vi "start_scanning.vi"(8 "error in (no error)":errorcluster, 11 "ScanModeDL090923Scaffold in":refnum<class "ImagingModeDL090923Scaffold.lvclass">) -> (0 "error out":errorcluster, 3 "ScanModeDL090923Scaffold out":refnum<class "ImagingModeDL090923Scaffold.lvclass">)   [LabVIEW 2010, in "ImagingModeDL090923Scaffold.lvclass"]
uses:
  ImagingModeDL090923Scaffold.lvclass
  ImagingModeDL090923Scaffold.lvclass/ImagingModeDL090923Scaffold.ctl
  common/classes/ErrorController/ErrorController/class_data.vi
  ScanHead/GenericScanHead/GenericScanHead/GenericScanHead.lvclass
  DAQ/GenericDAQ/GenericDAQ/GenericDAQ.lvclass
  common/classes/ErrorController/ErrorController/ErrorController.lvclass
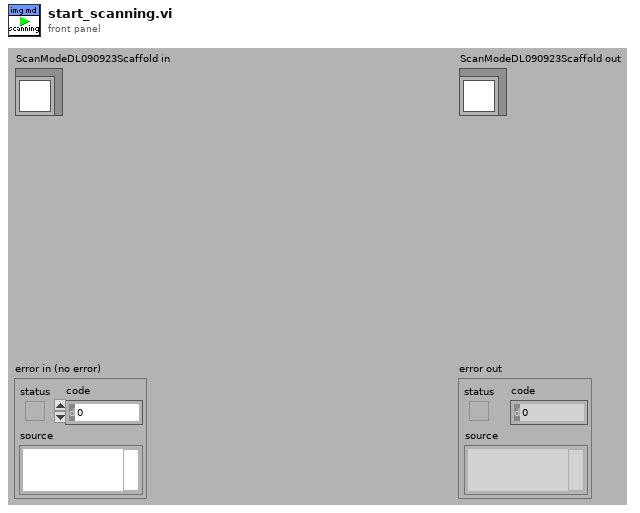
[diagram p1: front panel]
types:
  T1 = typedef "GenericToplevelComponent.lvclass/common_trigger_enum.ctl" = enum16{"NULL", "initialise", "terminate", "fetch command", "fetch data", "attach observer", "register as observer", "detach observer", "acknowledge", "start", "stop", "sweep started", "sweep finished", "experiment started", "experiment stopped"}
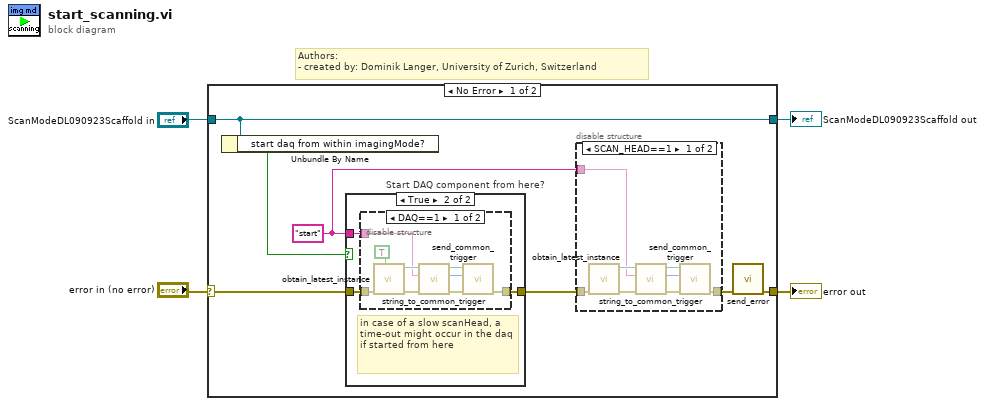
[diagram p0: block diagram]
diagram:
  # "Authors: \n- created by: Dominik Langer, University of Zurich, Switzerland"
  n1 = case shown="No Error" "error in (no error)" {
    selector: "error in (no error)" -> [w11 w36]
    tunnel: [w8 w36] -> w3
    tunnel: [w10 w35] -> w4
    tunnel: "ScanModeDL090923Scaffold in" -> [w10 w35]
    frame No Error {
      w5 = "start"
      n2 = Unbundle By Name(w10) -> ("start daq from within imagingMode?"=w9:bool)
      n3 = case "Start DAQ component from here?" shown="True" w9 {
        tunnel: [w12 w15] -> w6
        tunnel: w11 -> [w12 w14]
        tunnel: w5 -> [_ w13]
        frame False {
        }
        frame True {
          # "in case of a slow scanHead, a time-out might occur in the daq if started from here"
          n4 = disable-structure shown="DAQ==1" {
            disable-tunnel: w14 -> [w23 w25]
            disable-tunnel: [w24 w25] -> w15
            disable-tunnel: w13 -> [w18 _]
            frame condition #0 {
              n5 = call "obtain_latest_instance.vi"("quick, but maybe outdated?"=TRUE, "error in (no error)"=w23) -> ("error out"=w20:errorcluster, "GenericDAQ out"=w21:refnum<class "GenericDAQ.lvclass">)  [unwired: 8 out]
              n6 = call-dynamic "string_to_common_trigger.vi"("error in (no error)"=w20, "trigger string"=w18, "GenericToplevelComponent in"=w21) -> ("error out"=w19:errorcluster, "trigger"=w17:T1, "GenericToplevelComponent out"=w16:refnum<class "GenericDAQ.lvclass">)  [unwired: 6 in]
              n7 = call-dynamic "send_common_trigger.vi"("error in (no error)"=w19, "trigger"=w17, "GenericToplevelComponent in"=w16) -> ("error out"=w24:errorcluster)  [unwired: 6 in, 2 out]
            }
            frame condition #1 (active) {
            }
          }
        }
      }
      n8 = disable-structure shown="SCAN_HEAD==1" {
        disable-tunnel: w6 -> [w32 w34]
        disable-tunnel: [w33 w34] -> w7
        disable-tunnel: w5 -> [w26 _]
        frame condition #0 {
          n9 = call "obtain_latest_instance.vi"("error in (no error)"=w32) -> ("error out"=w31:errorcluster, "GenericScanHead out"=w29:refnum<class "GenericScanHead.lvclass">)  [unwired: 1 in, 8 out]
          n10 = call-dynamic "string_to_common_trigger.vi"("error in (no error)"=w31, "trigger string"=w26, "GenericToplevelComponent in"=w29) -> ("error out"=w30:errorcluster, "trigger"=w27:T1, "GenericToplevelComponent out"=w28:refnum<class "GenericScanHead.lvclass">)  [unwired: 6 in]
          n11 = call-dynamic "send_common_trigger.vi"("error in (no error)"=w30, "trigger"=w27, "GenericToplevelComponent in"=w28) -> ("error out"=w33:errorcluster)  [unwired: 6 in, 2 out]
        }
        frame condition #1 (active) {
        }
      }
      n12 = call "send_error.vi"("error in (no error)"=w7) -> ("error out"=w8:errorcluster)  [unwired: 10 in]
    }
    frame Error {
    }
  }
  "error out" <- w3
  "ScanModeDL090923Scaffold out" <- w4
